vi "Random in Range (Quad).vi"(1 "hi":i64, 4 "lo":i64) -> (6 "random":i64)   [LabVIEW 2021, in "EDT Numeric.lvlib"]
uses:
  EDT Numeric.lvlib
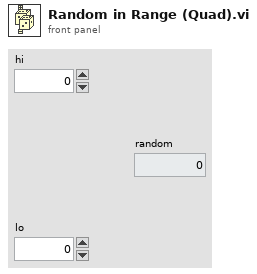
[diagram p1: front panel]
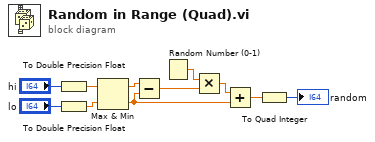
[diagram p0: block diagram]
diagram:
  n1 = To Double Precision Float(number="hi") -> (double precision float=w9:dbl)
  n2 = To Double Precision Float(number="lo") -> (double precision float=w8:dbl)
  n3 = Max & Min(x=w9, y=w8) -> (max(x,y)=w4:dbl, min(x,y)=w3:dbl)
  n4 = Subtract(x=w4, y=w3) -> (x-y=w6:dbl)
  n5 = Random Number (0-1)() -> (number: 0 to 1=w5:dbl)
  n6 = Multiply(x=w5, y=w6) -> (x*y=w7:dbl)
  n7 = Add(x=w7, y=w3) -> (x+y=w2:dbl)
  n8 = To Quad Integer(1:w2) -> (0:→"random":i64)
